vi "GetVIFromSubPanelByPathString.vi"(0 "VI Reference In":refnum<vi>, 2 "delimiter (>>)":string=">>", 5 "SubPanel Path":string, 11 "error in":errorcluster) -> (4 "VI Reference Out":refnum<vi>, 6 "SubPanel VI Reference":refnum<vi>, 15 "error out":errorcluster)   [LabVIEW 2016]
doc: "This VI gives the reference of the inserted VI in the SubPanel. \n\nThe SubPanel path input can be given with delimiters inbetween."
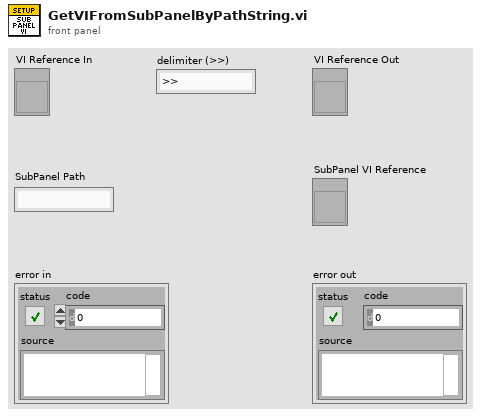
[diagram p1: front panel]
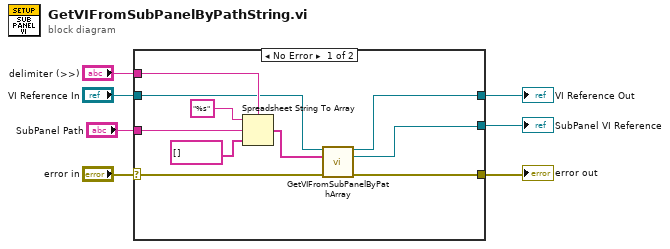
[diagram p0: block diagram]
diagram:
  n1 = case shown="No Error" "error in" {
    selector: "error in" -> [w12 w19]
    tunnel: "SubPanel Path" -> [w17 _]
    tunnel: "VI Reference In" -> [w11 w18]
    tunnel: [w9 w18] -> w4
    tunnel: [w13 w19] -> w3
    tunnel: "delimiter (>>)" -> [w14 _]
    tunnel: [w8 _] -> w1
    frame No Error {
      n2 = Spreadsheet String To Array(delimiter (Tab)=w14, format string="%s", spreadsheet string=w17, array type (2D Dbl)=string[] []) -> (array=w10:string[])
      n3 = call "GetVIFromSubPanelByPathArray.vi"("VI Reference in"=w11, "SubPanel Path"=w10, "error in (no error)"=w12) -> ("VI Reference out"=w9:refnum<vi>, "SubPanel VI Reference"=w8:refnum<vi>, "error out"=w13:errorcluster)  [unwired: 10 in]
    }
    frame Error {
    }
  }
  "error out" <- w3
  "VI Reference Out" <- w4
  "SubPanel VI Reference" <- w1
